vi "ReadBlockMod.vi"(0 "VISA Refnum in":refnum<visa-resource-name>, 1 "Command":string, 3 "error in (no error)":errorcluster) -> (7 "VISA Refnum out":refnum<visa-resource-name>, 8 "Read value":dbl, 10 "error out":errorcluster)   [LabVIEW 2023]
uses:
  <vilib>/regexp/Match Regular Expression.xnode
panel:
  out "String":string
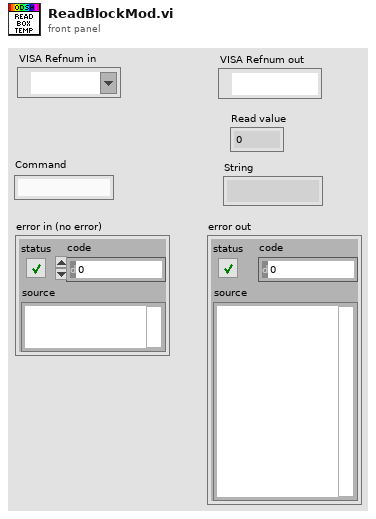
[diagram p1: front panel]
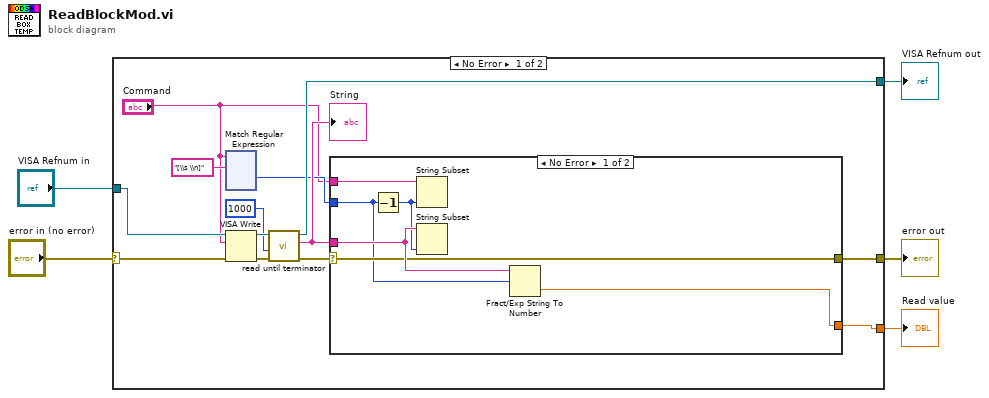
[diagram p0: block diagram]
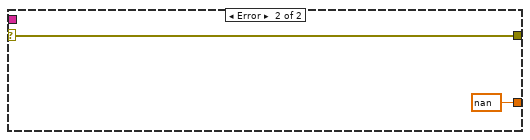
[diagram p2: hidden frame]
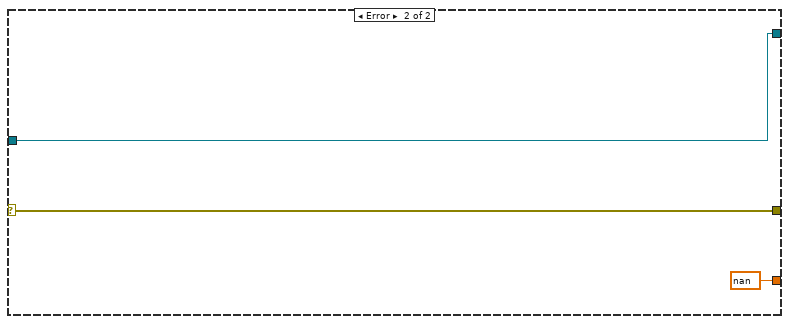
[diagram p3: hidden frame]
diagram:
  n1 = case shown="No Error" "error in (no error)" {
    selector: "error in (no error)" -> [w7 w146]
    tunnel: "VISA Refnum in" -> [w18 w145]
    tunnel: [w15 w145] -> w4
    tunnel: [w13 nan] -> w3
    tunnel: [w11 w146] -> w2
    frame No Error {
      n2 = xnode "Match Regular Expression"("chaîne en entrée"="Command", "expression régulière"="[\\s \\n]" ("regular expression")) -> ("offset après correspondance"=w8:i32)  [unwired: 4 in, 4 out]
      n3 = VISA Write(VISA resource name=w18, write buffer="Command", error in (no error)=w7) -> (VISA resource name out=w17:refnum<visa-resource-name>, error out=w16:errorcluster)  [unwired: 1 out]
      n4 = call "read until terminator.vi"("error in (no error)"=w16, "Timeout (ms)"=1000, "VISA Refnum in"=w17) -> ("error out"=w12:errorcluster, "String"=w10:string, "VISA Refnum out"=w15:refnum<visa-resource-name>)  [unwired: 6 in]
      "String" <- w10
      n5 = case shown="No Error" w12 {
        selector: w12 -> [w138 w142]
        tunnel: w10 -> [w139 _]
        tunnel: [w141 nan] -> w13
        tunnel: [w138 w142] -> w11
        tunnel: w8 -> [w137 _]
        tunnel: "Command" -> [w140 _]
        frame No Error {
          n6 = Decrement(x=w137) -> (x-1=w136:i32)
          n7 = String Subset(string=w140, length (rest)=w136) -> ()  [unwired: 1 in, 1 out]
          n8 = String Subset(string=w139, length (rest)=w136) -> ()  [unwired: 1 in, 1 out]
          n9 = Fract/Exp String To Number(string=w139, offset=w137) -> (number=w141:dbl)  [unwired: 2 in, 1 out]
        }
        frame Error {
        }
      }
    }
    frame Error {
    }
  }
  "error out" <- w2
  "VISA Refnum out" <- w4
  "Read value" <- w3
